vi "CookieGameLauncher.vi"   [LabVIEW 2020]
types:
  T1 = enum32{"Invalid", "Standard", "Closed", "Hidden", "Minimized", "Maximized"}
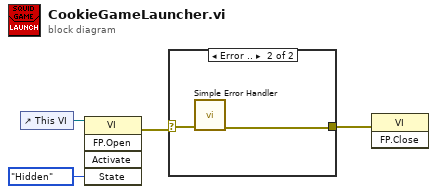
[diagram p0: block diagram]
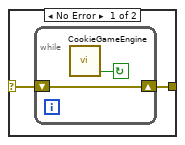
[diagram p2: hidden frame]
diagram:
  n1 = control-ref of="This VI"() -> (w4:refnum<vi>)
  n2 = invoke class="VI" method="FP.Open"(reference=w4, "State"=T1."Hidden") -> (error out=w2:errorcluster)  [unwired: 3 in, 4 out]
  n3 = case shown="Error .." w2 {
    selector: w2 -> [w6 w10]
    tunnel: [w5 w9] -> w1
    frame No Error {
      n4 = while {
        shift-right: [w7] -> w5
        shift-left: w6 -> [w7]
        stop <- w8 continue-if-true
        n5 = call "CookieGameEngine.vi"() -> ("PlayAgain"=w8:bool)  [unwired: 5 in]
      }
    }
    frame Error {
      n6 = call <vilib>:"Simple Error Handler.vi"("error in (no error)"=w10) -> ("error out"=w9:errorcluster)  [unwired: 4 in, 4 out]
    }
  }
  n7 = invoke class="VI" method="FP.Close"(error in=w1) -> ()  [unwired: 2 in, 3 out]
